vi "Auto Aim.vi"(5 "Turning Angle":dbl, 7 "RobotDriveDevRef in":T1, 8 "Angle robot facing":dbl, 9 "Target Boundries":cluster{"Upper":dbl, "Lower":dbl}) -> ()   [LabVIEW 2017]
uses:
  <vilib>/Rock Robotics/WPI/RobotDrive/WPI_RobotDriveDevRef.ctl
  <vilib>/Rock Robotics/WPI/MotorControl/WPI_MotorControlDeviceRef.ctl
  <vilib>/Rock Robotics/WPI/MotorControl/WPI_MotorControlType.ctl
  <vilib>/Rock Robotics/SystemInterfaces/DIO/FPGA_DIOPWMChannel.ctl
  <vilib>/Rock Robotics/WPI/PWM/WPI_PWMDeadband.ctl
  <vilib>/Rock Robotics/SystemInterfaces/DIO/FPGA_DIOChannel.ctl
  <vilib>/Rock Robotics/WPI/Utilities/WPI_GetSetVariantRefNum.vi
  <vilib>/Rock Robotics/Network Tables/NT Read Number.vi
  <vilib>/Rock Robotics/WPI/RobotDrive/WPI_RobotDriveArcadeDrive_Standard(NoSaturation).vi
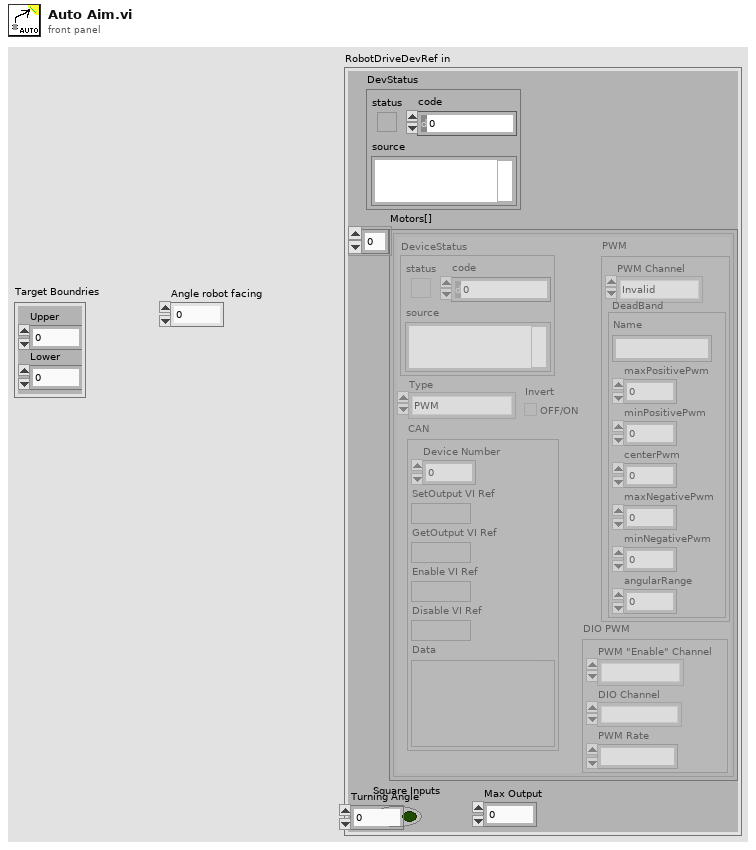
[diagram p1: front panel]
types:
  T1 = typedef "WPI_RobotDriveDevRef.ctl" = cluster{"DevStatus":errorcluster, "Motors[]":T2[], "Square Inputs":bool, "Max Output":dbl}
  T2 = typedef "WPI_MotorControlDeviceRef.ctl" = cluster{"DeviceStatus":errorcluster, "Type":T3, "PWM":cluster{"PWM Channel":T4, "DeadBand":T5}, "CAN":cluster{"Device Number":u8, "SetOutput VI Ref":variant, "GetOutput VI Ref":variant, "Enable VI Ref":variant, "Disable VI Ref":variant, "Data":variant}, "Invert":bool, "DIO PWM":cluster{"PWM \"Enable\" Channel":T4, "DIOChannel":T6, "PWM Rate":dbl}}
  T3 = typedef "WPI_MotorControlType.ctl" = enum16{"PWM", "CAN", "DIO PWM"}
  T4 = typedef "FPGA_DIOPWMChannel.ctl" = enum8{"PWM 0", "PWM 1", "PWM 2", "PWM 3", "PWM 4", "PWM 5", "PWM 6", "PWM 7", "PWM 8", "PWM 9", "PWM MXP 0", "PWM MXP 1", "PWM MXP 2", "PWM MXP 3", "PWM MXP 4", "PWM MXP 5", "PWM MXP 6", "PWM MXP 7", "PWM MXP 8", "PWM MXP 9", "Invalid"}
  T5 = typedef "WPI_PWMDeadband.ctl" = cluster{"Name":string, "maxPositivePwm":i32, "minPositivePwm":i32, "centerPwm":i32, "maxNegativePwm":i32, "minNegativePwm":i32, "angularRange":u16}
  T6 = typedef "FPGA_DIOChannel.ctl" = enum8{"DIO 0", "DIO 1", "DIO 2", "DIO 3", "DIO 4", "DIO 5", "DIO 6", "DIO 7", "DIO 8", "DIO 9", "DIO MXP 0", "DIO MXP 1", "DIO MXP 2", "DIO MXP 3", "DIO MXP 4", "DIO MXP 5", "DIO MXP 6", "DIO MXP 7", "DIO MXP 8", "DIO MXP 9", "DIO MXP 10", "DIO MXP 11", "DIO MXP 12", "DIO MXP 13", "DIO MXP 14", "DIO MXP 15", "SPI Port CS1", "SPI Port CS2", "SPI Port CS3", "SPI Port MISO", "SPI Port MOSI", "Invalid"}
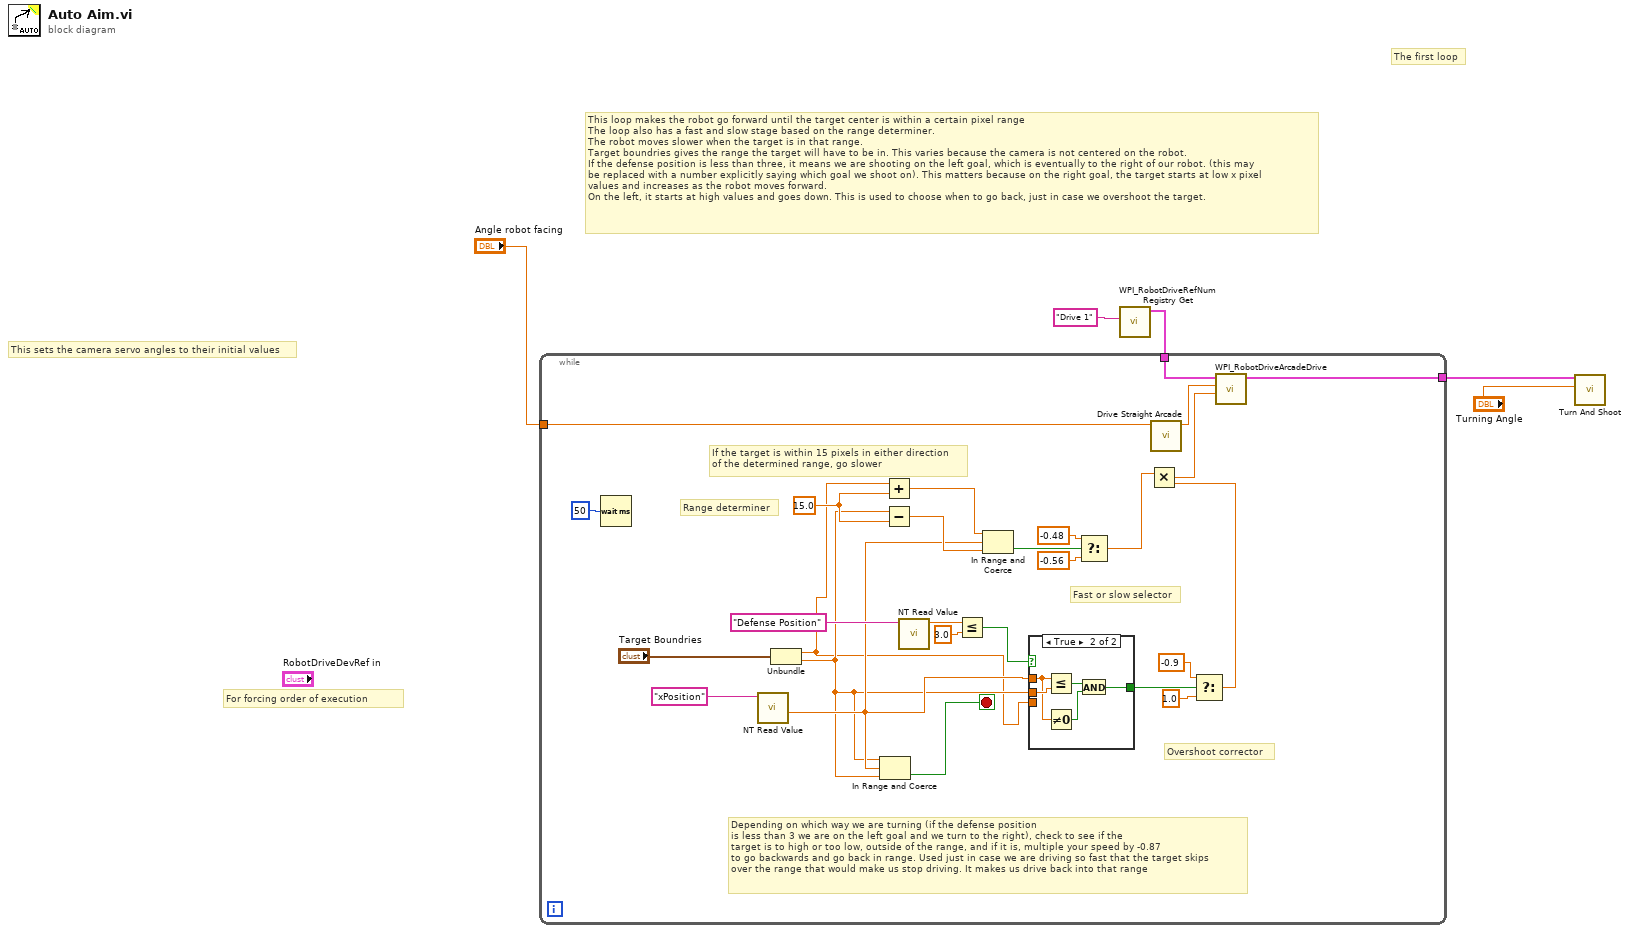
[diagram p0: block diagram]
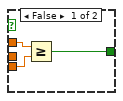
[diagram p2: hidden frame]
diagram:
  # "This loop makes the robot go forward until the target center is within a certain pixel range\nThe loop also has a fast and slow stage based on the range determiner.\nThe robot moves slower when the target is in that range.\nTarget boundries gives the range the target will have to be in. This varies because the camera is not centered on the robot.\nIf the defense position is less than three, it means we are shooting on the left goal, which is eventually to the right of our robot. (this may \nbe replaced with a number explicitly saying which goal we shoot on). This matters because on the right goal, the target starts at low x pixel \nvalues and increases as the robot moves forward.\nOn the left, it starts at high values and goes down. This is used to choose when to go back, just in case we overshoot the target."
  # "The first loop"
  # "This sets the camera servo angles to their initial values"
  # "For forcing order of execution"
  n1 = call <vilib>:"WPI_RobotDriveRefNum Registry Get.vi"("refnum name"="Drive 1") -> ("RobotDriveDevRef"=w2:T1)  [unwired: 9 in, 1 out]
  n2 = while {
    tunnel: [w30] -> w1
    tunnel: "Angle robot facing" -> [w21]
    tunnel: w2 -> [w11]
    stop <- w29 stop-if-true
    w23 = 15.0 ("y")
    # "If the target is within 15 pixels in either direction \nof the determined range, go slower"
    # "Depending on which way we are turning (if the defense position \nis less than 3 we are on the left goal and we turn to the right), check to see if the\ntarget is to high or too low, outside of the range, and if it is, multiple your speed by -0.87\nto go backwards and go back in range. Used just in case we are driving so fast that the target skips\nover the range that would make us stop driving. It makes us drive back into that range"
    # "Overshoot corrector"
    # "Fast or slow selector"
    # "Range determiner"
    n3 = Wait (ms)(milliseconds to wait=u32 50) -> ()  [unwired: 1 out]
    n4 = call-poly <vilib>:"NT Read Value.vi"("Name"="xPosition") -> ("Numeric"=w8:dbl)  [unwired: 9 in, 1 out]
    n5 = Unbundle("Target Boundries") -> ("Upper"=w6:dbl, "Lower"=w7:dbl)
    n6 = In Range and Coerce(upper limit=w7, x=w8, lower limit=w7) -> (In Range?=w29:bool)  [unwired: 1 out]
    n7 = Add(x=w6, y=w23) -> (x+y=w24:dbl)
    n8 = Subtract(x=w7, y=w23) -> (x-y=w16:dbl)
    n9 = call-poly <vilib>:"NT Read Value.vi"("Name"="Defense Position") -> ("Numeric"=w14:dbl)  [unwired: 9 in, 1 out]
    n10 = Less Or Equal?(x=w14, y=3.0) -> (x <= y?=w10:bool)
    n11 = In Range and Coerce(upper limit=w24, x=w8, lower limit=w16) -> (In Range?=w28:bool)  [unwired: 1 out]
    n12 = case shown="True" w10 {
      tunnel: w8 -> [w35 w37]
      tunnel: w7 -> [_ w38]
      tunnel: [w34 w36] -> w9
      tunnel: w6 -> [w33 _]
      frame False {
        n13 = Greater Or Equal?(x=w35, y=w33) -> (x >= y?=w34:bool)
      }
      frame True {
        n14 = Less Or Equal?(x=w37, y=w38) -> (x <= y?=w40:bool)
        n15 = Not Equal To 0?(x=w37) -> (x != 0?=w39:bool)
        n16 = And(x=w40, y=w39) -> (x .and. y?=w36:bool)
      }
    }
    n17 = Select(t=-0.48 ("Y axis value"), s=w28, f=-0.56 ("Y axis value")) -> (s? t:f=w18:dbl)
    n18 = call "Drive Straight Arcade.vi"("Angle robot facing"=w21) -> ("Arcade drive x"=w22:dbl)  [unwired: 10 in]
    n19 = Select(t=-0.9, s=w9, f=1.0) -> (s? t:f=w12:dbl)
    n20 = Multiply(x=w18, y=w12) -> (x*y=w17:dbl)
    n21 = call-poly <vilib>:"WPI_RobotDriveArcadeDrive.vi"("Y axis value"=w17, "X axis value"=w22, "RobotDriveDevRef"=w11) -> ("RobotDriveDevRef"=w30:T1)  [unwired: 6 in, 2 out]
  }
  n22 = call "Turn And Shoot.vi"("Turning Angle"="Turning Angle", "RobotDriveDevRef"=w1) -> ()  [unwired: 10 in]
